vi "Right Gripper Close.vi"(6 "Delay":u32=500, 8 "Target Position":sgl, 9 "Threshold":sgl=10.0, 10 "Pause on Miss?":bool, 11 "error in":errorcluster) -> (0 "On Target":bool, 3 "error out":errorcluster)   [LabVIEW 2013]
uses:
  ROS/Code/SubVIs/BaxterSide.ctl
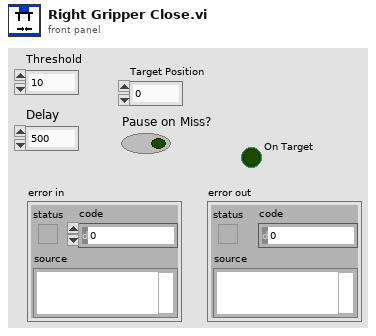
[diagram p1: front panel]
types:
  T1 = typedef "BaxterSide.ctl" = enum16{"left", "right"}
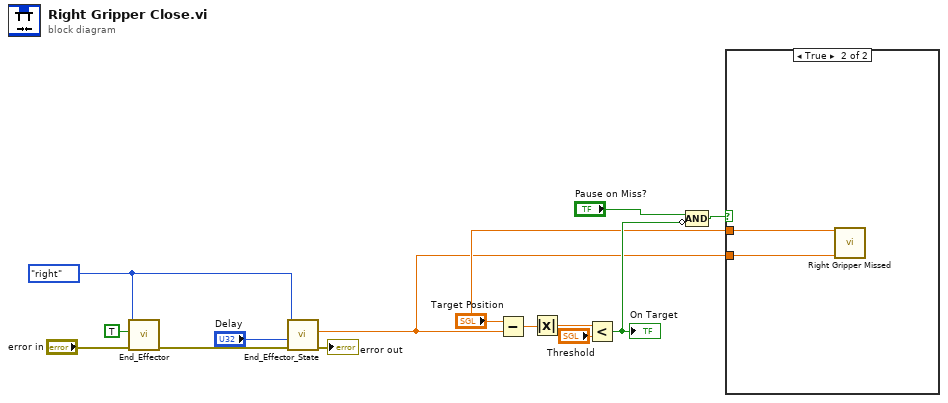
[diagram p0: block diagram]
diagram:
  w7 = BaxterSide."right" ("Side")
  n1 = call "End_Effector.vi"("error in"="error in", "Close"=TRUE, "Side"=w7) -> ("error out"=w14:errorcluster)  [unwired: 5 in]
  n2 = call "End_Effector_State.vi"("error in"=w14, "Delay"="Delay", "Side"=w7) -> ("error out"=→"error out":errorcluster, "position"=w1:sgl)  [unwired: 2 in, 2 out]
  n3 = Subtract(x="Target Position", y=w1) -> (x-y=w11:sgl)
  n4 = Absolute Value(x=w11) -> (abs(x)=w10:sgl)
  n5 = Less?(x=w10, y="Threshold") -> (x < y?=w4:bool)
  "On Target" <- w4
  n6 = Compound Arithmetic op=AND("Pause on Miss?", invert w4) -> (w5:bool)
  n7 = case shown="True" w5 {
    tunnel: "Target Position" -> [_ w16]
    tunnel: w1 -> [_ w15]
    frame False {
    }
    frame True {
      n8 = call "Right Gripper Missed.vi"("Gripper Opening"=w15, "Object Size"=w16) -> ()  [unwired: 8 in]
    }
  }
